vi "EncodeUInt8.vi"(1 "Data In":u8[](array[numeric])) -> (0 "Data Out":u8[](array[numeric]))   [LabVIEW 2015, in "navX Library v1 (deprecated).lvlib"]
uses:
  navX Library v1 (deprecated).lvlib
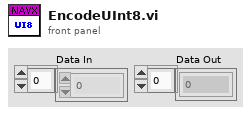
[diagram p1: front panel]
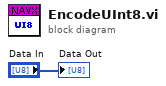
[diagram p0: block diagram]
diagram:
  "Data Out" <- "Data In"
